vi "Maui.Config.WriteSpecificConfigPath.vi"(8 "error in (no error)":errorcluster, 10 "Specific Configuration":path, 11 "Maui.Config in":refnum<class "Maui.Config.lvclass">) -> (0 "error out":errorcluster, 3 "Maui.Config out":refnum<class "Maui.Config.lvclass">)   [LabVIEW 2019, in "Maui.Config.lvclass"]
uses:
  Maui.Config.lvclass
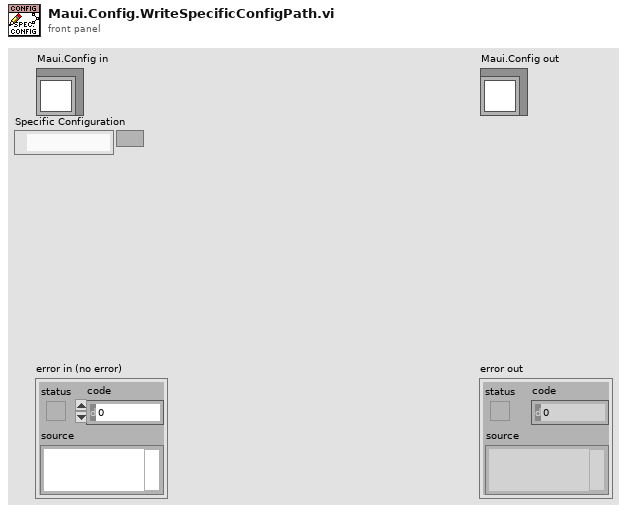
[diagram p1: front panel]
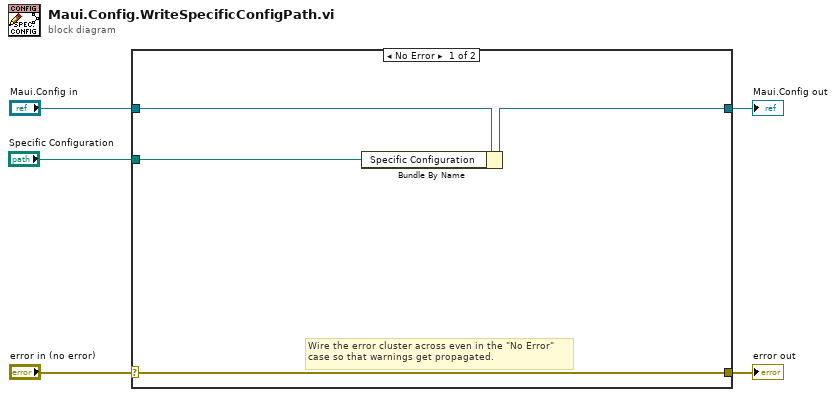
[diagram p0: block diagram]
diagram:
  n1 = case shown="No Error" "error in (no error)" {
    selector: "error in (no error)" -> [w8 w11]
    tunnel: [w8 w11] -> w4
    tunnel: [w7 w10] -> w2
    tunnel: "Maui.Config in" -> [w9 w10]
    tunnel: "Specific Configuration" -> [w6 _]
    frame No Error {
      # "Wire the error cluster across even in the \"No Error\"\ncase so that warnings get propagated."
      n2 = Bundle By Name(cluster=w9, "Specific Configuration"=w6) -> (w7:refnum<class "Maui.Config.lvclass">)
    }
    frame Error {
    }
  }
  "error out" <- w4
  "Maui.Config out" <- w2
